vi "SlackAPI-chat.postMessage.vi"(0 "access_token":string, 5 "user ID":string, 7 "message":string, 9 "username":string, 11 "error in (no error)":errorcluster) -> (15 "error out":errorcluster)   [LabVIEW 2020]
uses:
  SlackAPI-chat.postMessage Cluster.ctl
  <vilib>/httpClient/POSTBuffer.vi
  <vilib>/httpClient/LabVIEWHTTPClient.lvlib
panel:
  out "headers":string
  out "body":string
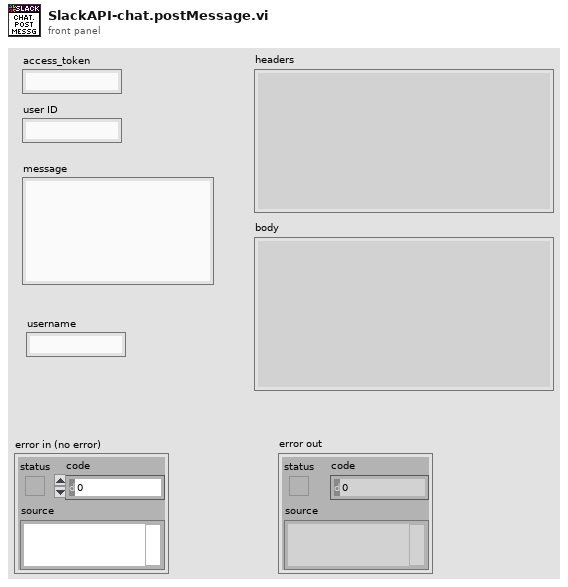
[diagram p1: front panel]
types:
  T1 = typedef "SlackAPI-chat.postMessage Cluster.ctl" = cluster{"token":string, "channel":string, "text":string, "username":string}
  T2 = typedef "LabVIEWHTTPClient.lvlib/ClientHandle.ctl" = refnum<k1>
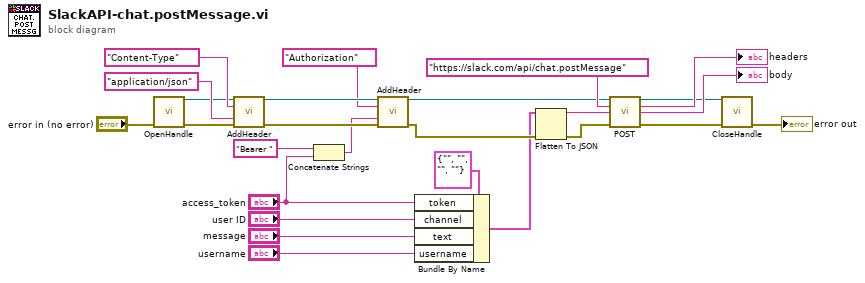
[diagram p0: block diagram]
diagram:
  n1 = call <vilib>:"OpenHandle.vi"("error in (no error)"="error in (no error)") -> ("client handle out"=w19:T2, "error out"=w15:errorcluster)  [unwired: 13 in]
  n2 = call <vilib>:"AddHeader.vi"("client handle"=w19, "header"="Content-Type", "value"="application/json", "error in (no error)"=w15) -> ("client handle out"=w17:T2, "error out"=w16:errorcluster)  [unwired: 10 in]
  n3 = Concatenate Strings("Bearer " ("string"), "access_token") -> (w13:string)
  n4 = call <vilib>:"AddHeader.vi"("client handle"=w17, "header"="Authorization", "value"=w13, "error in (no error)"=w16) -> ("client handle out"=w18:T2, "error out"=w11:errorcluster)  [unwired: 10 in]
  n5 = Bundle By Name(cluster=T1 {"token"="", "channel"="", "text"="", "username"=""} ("postMessageCluster"), "token"="access_token", "channel"="user ID", "text"="message", "username"="username") -> (w2:T1)
  n6 = Flatten To JSON(anything=w2, error in (no error)=w11) -> (JSON string=w23:string, 11:w22:errorcluster)  [unwired: 1 in]
  n7 = call-poly <vilib>:"POST.vi"("client handle"=w18, "url"="https://slack.com/api/chat.postMessage", "buffer"=w23, "error in (no error)"=w22) -> ("client handle out"=w9:T2, "headers"=→"headers":string, "body"=→"body":string, "error out"=w8:errorcluster)  [unwired: 8 in]
  n8 = call <vilib>:"CloseHandle.vi"("client handle"=w9, "error in (no error)"=w8) -> ("error out"=→"error out":errorcluster)  [unwired: 13 in]
